vi "DELETEME.vi"() -> ()   [LabVIEW 2024]
uses:
  <vilib>/Utility/Data Type/Type Definitions/Data Type.ctl
  tests/MyEventGrid/MyEventGrid.lvclass
  tests/MyEventGrid/MyEventGrid.lvclass/MyEventGrid.ctl
  Cells/Cell Context/Cell Context.lvclass
  SourceGrid.lvclass
  <vilib>/Utility/Data Type/NI_Data Type.lvlib
  D:/git/Sourcegrid-LabVIEW/source/Grid/SourceGrid.lvclass
  D:/git/Sourcegrid-LabVIEW/tests/MyEventGrid/MyEventGrid.lvclass
  D:/git/Sourcegrid-LabVIEW/dll/SourceGrid.dll
  dll/SourceGrid.dll
panel:
  out "onClick Value":variant
  out "onValueChanged Value type":T1
  out "onValueChanged Value":variant
  out "error out":errorcluster
  in  "Grid Container":refnum<k24>(container)
  in  "stop":bool
  out "onClick Position":string
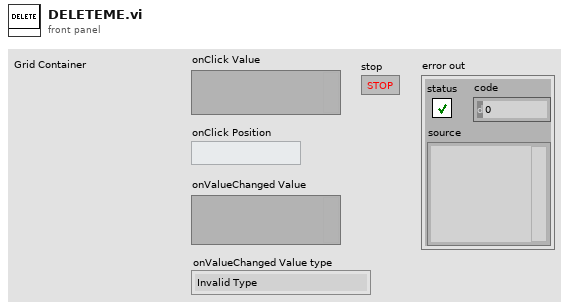
[diagram p1: front panel]
types:
  T1 = typedef "NI_Data Type.lvlib/Data Type.ctl" = enum8{"Invalid Type", "Void", "I8", "I16", "I32", "I64", "U8", "U16", "U32", "U64", "Single Float", "Double Float", "Extended Float", "Single Complex", "Double Complex", "Extended Complex", "Enum U8", "Enum U16", "Enum U32", "Enum U64", "Single Float With Unit", "Double Float With Unit", "Extended Float With Unit", "Single Complex with Unit", "Double Complex with Unit", "Extended Complex with Unit", "Boolean", "String", "Path", "Picture", "Tag", "Array", "Cluster", "Variant", "LV Variant", "Waveform", "Timestamp", "Digital Waveform", "Digital Data", "ExpressData", "Refnum", "External Data", "VI", "Poly VI", "LabVIEW Class Instance", "Fixed Point", "Set Collection", "Map Collection"}
  T2 = cluster{"onClick":refnum<user-event>, "onDoubleClick":refnum<user-event>, "onValueChanged":refnum<user-event>}
  T3 = typedef "Rendezvous RefNum" = refnum<k1>
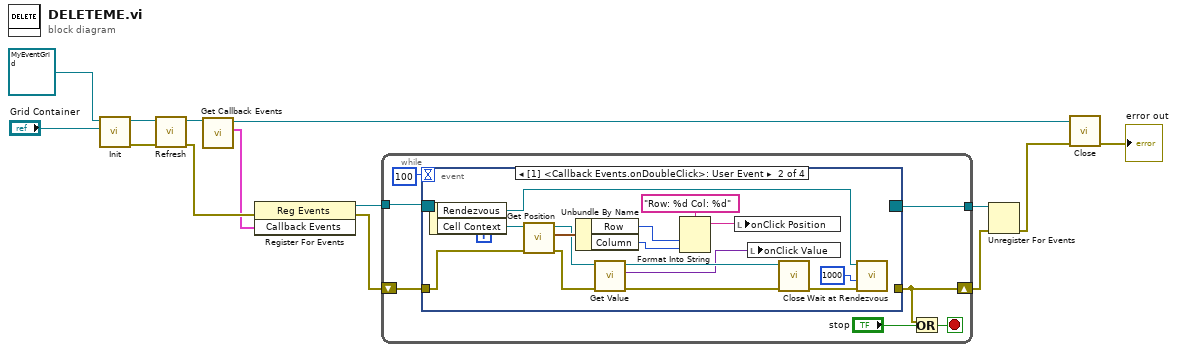
[diagram p0: block diagram]
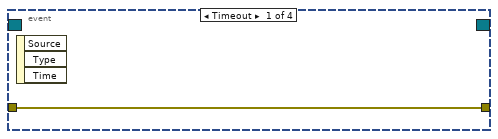
[diagram p2: hidden frame]
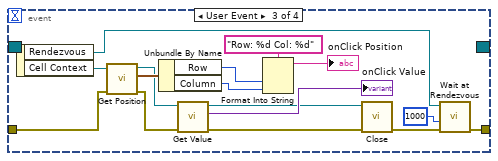
[diagram p3: hidden frame]
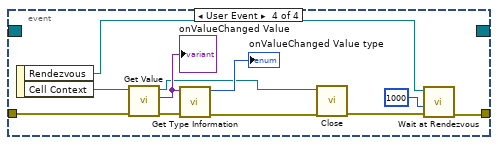
[diagram p4: hidden frame]
diagram:
  n1 = call-dynamic "Init.vi"("Sourcegrid Container"="Grid Container", "MyEventGrid in"=refnum<class "MyEventGrid.lvclass"> refnum ("Grid in")) -> ("error out"=w10:errorcluster, "MyEventGrid out"=w9:refnum<class "MyEventGrid.lvclass">)  [unwired: 8 in]
  n2 = call "Refresh.vi"("error in"=w10, "SourceGrid in"=w9) -> ("error out"=w11:errorcluster, "SourceGrid out"=w8:refnum<class "MyEventGrid.lvclass">)  [unwired: 8 in]
  n3 = call "Get Callback Events.vi"("MyEventGrid in"=w8) -> ("Callback Events"=w6:T2, "MyEventGrid out"=w7:refnum<class "MyEventGrid.lvclass">)  [unwired: 9 in]
  n4 = register-events(error in=w11, w6) -> (reference out=w3:refnum<event-registration>, error out=w2:errorcluster)  [unwired: 1 in]
  n5 = while {
    tunnel: w3 -> [w20]
    tunnel: [w19] -> w4
    shift-right: [w16] -> w1
    shift-left: w2 -> [w15]
    stop <- w17 stop-if-true
    n6 = event shown="[1] <Callback Events.onDoubleClick>: User Event" {
      selector: w20 -> [_ _ _ _]
      dyn-events: [_ _ _ _] -> w19
      timeout: 100 -> [_ _ _ _]
      tunnel: [w22 _ w43 w57] -> w16
      tunnel: w15 -> [w22 w26 w46 w63]
      event Timeout {
        n7 = event-data() -> ()  [unwired: 1 in, 3 out]
      }
      event User Event {
        n8 = event-data() -> ("Rendezvous"=w23:T3, "Cell Context"=w27:refnum<class "Cell Context.lvclass">)  [unwired: 1 in]
        n9 = call "Get Position.vi"("error in"=w26, "Cell Context in"=w27) -> ("error out"=w33:errorcluster, "Position"=w37:cluster{"Row":i32, "Column":i32}, "Cell Context out"=w32:refnum<class "Cell Context.lvclass">)  [unwired: 7 in]
        n10 = Unbundle By Name(w37) -> ("Row"=w35:i32, "Column"=w34:i32)
        n11 = call "Get Value.vi"("error in (no error)"=w33, "Cell Context in"=w32) -> ("error out"=w31:errorcluster, "Value"=w25:variant, "Cell Context out"=w28:refnum<class "Cell Context.lvclass">)  [unwired: 7 in]
        n12 = Format Into String(format string="Row: %d Col: %d", w35, w34) -> (resulting string=w24:string)  [unwired: 2 in, 1 out]
        n13 = local write "onClick Position"(w24) -> ()
        n14 = local write "onClick Value"(w25) -> ()
        n15 = call "Close.vi"("error in"=w31, "Cell Context in"=w28) -> ("error out"=w29:errorcluster)  [unwired: 8 in, 1 out]
        n16 = call <vilib>:"Wait at Rendezvous.vi"("error in (no error)"=w29, "ms timeout (-1)"=1000, "rendezvous"=w23) -> ()  [unwired: 2 in, 3 out]
      }
      event User Event {
        n17 = event-data() -> ("Rendezvous"=w42:T3, "Cell Context"=w53:refnum<class "Cell Context.lvclass">)  [unwired: 1 in]
        n18 = call "Get Position.vi"("error in"=w46, "Cell Context in"=w53) -> ("error out"=w47:errorcluster, "Position"=w52:cluster{"Row":i32, "Column":i32}, "Cell Context out"=w45:refnum<class "Cell Context.lvclass">)  [unwired: 7 in]
        n19 = Unbundle By Name(w52) -> ("Row"=w49:i32, "Column"=w48:i32)
        n20 = call "Get Value.vi"("error in (no error)"=w47, "Cell Context in"=w45) -> ("error out"=w41:errorcluster, "Value"=→"onClick Value":variant, "Cell Context out"=w38:refnum<class "Cell Context.lvclass">)  [unwired: 7 in]
        n21 = Format Into String(format string="Row: %d Col: %d", w49, w48) -> (resulting string=→"onClick Position":string)  [unwired: 2 in, 1 out]
        n22 = call "Close.vi"("error in"=w41, "Cell Context in"=w38) -> ("error out"=w39:errorcluster)  [unwired: 8 in, 1 out]
        n23 = call <vilib>:"Wait at Rendezvous.vi"("error in (no error)"=w39, "ms timeout (-1)"=1000, "rendezvous"=w42) -> ("error out"=w43:errorcluster)  [unwired: 2 in, 2 out]
      }
      event User Event {
        n24 = event-data() -> ("Rendezvous"=w59:T3, "Cell Context"=w64:refnum<class "Cell Context.lvclass">)  [unwired: 1 in]
        n25 = call "Get Value.vi"("error in (no error)"=w63, "Cell Context in"=w64) -> ("error out"=w61:errorcluster, "Value"=w62:variant, "Cell Context out"=w54:refnum<class "Cell Context.lvclass">)  [unwired: 7 in]
        "onValueChanged Value" <- w62
        n26 = call <vilib>:"Get Type Information.vi"("error in (no error)"=w61, "variant"=w62) -> ("error out"=w56:errorcluster, "type"=→"onValueChanged Value type":T1)  [unwired: 5 in, 3 out]
        n27 = call "Close.vi"("error in"=w56, "Cell Context in"=w54) -> ("error out"=w55:errorcluster)  [unwired: 8 in, 1 out]
        n28 = call <vilib>:"Wait at Rendezvous.vi"("error in (no error)"=w55, "ms timeout (-1)"=1000, "rendezvous"=w59) -> ("error out"=w57:errorcluster)  [unwired: 2 in, 2 out]
      }
    }
    n29 = Or(x=w16, y="stop") -> (x .or. y?=w17:bool)
  }
  n30 = Unregister For Events(event registration refnum=w4, error in=w1) -> (error out=w12:errorcluster)
  n31 = call-dynamic "Close.vi"("error in"=w12, "MyEventGrid in"=w7) -> ("error out"=→"error out":errorcluster)  [unwired: 8 in, 1 out]
